vi "tcp_client_microwave.vi"(0 "conn_id_in":refnum<k5>, 5 "addr":string="192.168.24.191", 7 "port":u16=10000, 11 "error in":errorcluster) -> (4 "conn_id_out":refnum<k5>, 6 "Raw data array":string[](array[string]), 8 "event_num":i32, 10 "pol":dbl, 15 "error out":errorcluster)   [LabVIEW 2019]
panel:
  out "status":bool
  in  "stop":bool
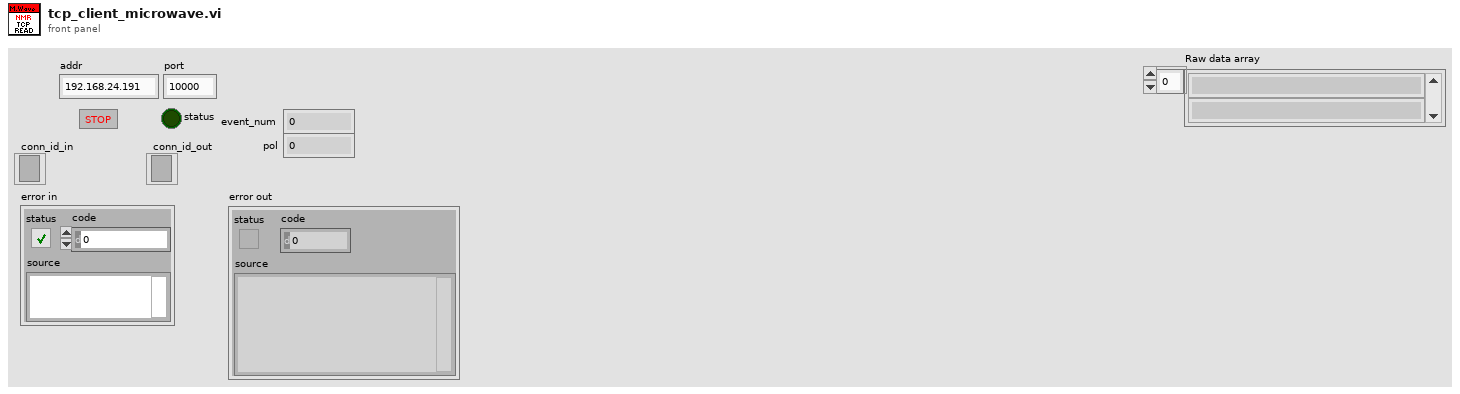
[diagram p1: front panel]
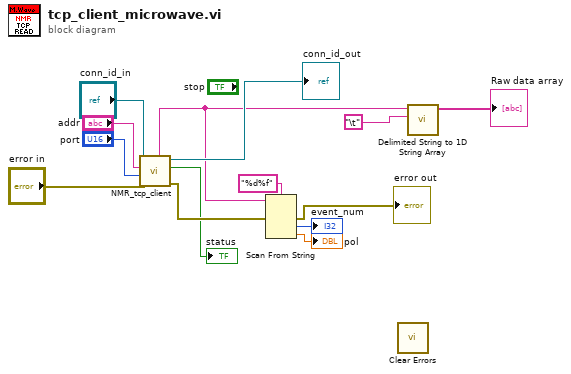
[diagram p0: block diagram]
diagram:
  n1 = call "NMR_tcp_client.vi"("error in"="error in", "port"="port", "address"="addr", "conn_id_in"="conn_id_in") -> ("error out"=w12:errorcluster, "status"=→"status":bool, "conn_id_out"=→"conn_id_out":refnum<k5>, "data out"=w1:string)  [unwired: 3 in, 1 out]
  n2 = Scan From String(format string="%d%f", input string=w1, error in=w12) -> (error out=→"error out":errorcluster, output 1=→"event_num":i32, output 2=→"pol":dbl)  [unwired: 3 in, 2 out]
  n3 = call <vilib>:"Clear Errors.vi"() -> ()  [unwired: 6 in, 2 out]
  n4 = call <vilib>:"Delimited String to 1D String Array.vi"("delimiter"="\t", "delimited string"=w1) -> ("string array"=→"Raw data array":string[])  [unwired: 9 in]
